vi "Configure.vi"(0 "disk streaming in":refnum<class "Disk Streaming.lvclass">, 1 "actual host DMA buffer size (samples)":u32, 2 "actual host DMA buffer size (elements)":u32, 3 "transfer quantum size (samples)":u64, 4 "sample count (-1)":i64=-1, 5 "error in (no error)":errorcluster, 6 "coerce sample count? (T)":bool=TRUE, 7 "reserve file size (F)":bool, 8 "record count (1)":i64=1, 9 "max operations":u32, 11 "timeout (5 s)":dbl=5.0) -> (13 "actual max operations":u32, 14 "disk streaming out":refnum<class "Disk Streaming.lvclass">, 15 "file allocation size (bytes)":u64, 16 "file size (samples)":i64, 18 "sample count out":i64, 19 "error out":errorcluster)   [LabVIEW 2021, in "Disk Streaming.lvclass"]
doc: "Configures the transfer parameters of the streaming between a disk and an FPGA Target. Open a TDMS file and create a disk streaming instance referencing the file for streaming samples between a disk and an FPGA Target using the <B>Open.vi</B>, then use this VI to configure the transfer. Use the <B>Get Next Transfer Size.vi</B> to get the size of the next block to transfer during the streaming process, then depending on the selected direction and the TDMS I/O functions, use the <B>Read (I16 Data Ref).vi</B>, <B>Read (I16).vi</B>, <B>Write (I16 Data Ref).vi</B> or <B>Write (I16).vi</B> to read or write the TDMS file. Use the <B>Configure Status.vi</B> to configure the streaming status properties. Use the <B>Get Status.vi</B> to get status information. Use the <B>Close.vi</B> to close the disk streaming instance and the TDMS file it uses.\n\nInputs:\n\n<B>disk streaming in</B>: Disk streaming instance input.\n\n<B>actual host DMA buffer size (samples)</B>: The size, in number of samples, of the host DMA buffer transferring the samples between the host and the FPGA Target.\n\n<B>actual host DMA buffer size (elements)</B>: The size, in number of elements, of the host DMA buffer transferring the samples between the host and the FPGA Target.\n\n<B>transfer quantum size (samples)</B>: The quantum size, in number of samples, supported by the FPGA Target when transferring samples between the host and the FPGA Target. The number of samples transferred in each block during the streaming is a multiple of this value.\n\n<B>sample count</B>, <B>record count</B>: The number of samples per record and the number of records to transfer during the streaming. Set any of these inputs to -1 for infinite streaming. When streaming to disk, use non-negative values on these inputs to configure a finite streaming to stream <B>record count</B> * <B>sample count</B> number of samples to disk. Similarly, when streaming from disk, a non-zero <B>sample count</B> value configures a finite streaming to stream <B>record count</B> * <B>sample count</B> samples from disk. When the end of file is reached during a stream from disk process, the file is reopened, and the file reading continues from the beginning of the file. When streaming from disk, a zero <B>sample count</B> value configures a finite streaming to stream until the end of file is reached <B>record count</B> times. The default value of the <B>sample count</B> input is -1, while the default value of the <B>record count</B> input is 1.\n\n<B>coerce sample count?</B>: If this input is true, then the <B>sample count</B> input will be rounded up to be a multiple of the device transfer quantum size and the disk transfer quantum size. The rounded value is returned on the <B>sample count out</B> output, and the VI will use the rounded value as the number of samples per record. The default value of this input is true.\n\n<B>reserve file size</B>: Set this input to true when streaming to disk to pre-allocate disk space for the TDMS file and to prevent fragmentation on a file-system level. The pre-allocation is only possible when performing a finite streaming to disk, otherwise this input is ignored. Note: on Windows systems with the User Account Control enabled the file pre-allocation requires to run LabVIEW or the application with administrator privileges to avoid a run-time error. The default value of this input is false.\n\n<B>max operations</B>: The maximum number of asynchronous reads or writes that can run simultaneously in the background. This VI uses an upper limit for this parameter which is the number of blocks that can fit into the host DMA buffer minus 1 (the value used on the <B># of blocks</B> input of the <B>Disk Streaming Open.vi</B> minus 1). If this input is less than 1, then the upper limit value is used instead, otherwise the value of this input is coerced between 1 and the upper limit. The default value of this input is 0.\n\n<B>timeout</B>: The timeout value, in seconds, for the TDMS asynchronous read or write functions. When the number of pending asynchronous operations reaches the maximum value, the TDMS asynchronous read or write function waits as long as the timeout value for a pending asynchronous operation to complete before issuing another asynchronous operation. If no asynchronous operation completes during the wait period, then the function returns a timeout error. The default value of this input is 5.\n\nOutputs:\n\n<B>disk streaming out</B>: Disk streaming instance output. Pass this output to the other Disk Streaming VIs to perform the streaming.\n\n<B>file allocation size (bytes)</B>: The number of bytes pre-allocated for the TDMS file. For large files of several terabytes, the operating system may take a significant amount of time to pre-allocate disk space. Insert a delay in your application after this VI to ensure the file size is fully reserved. For multiple files on separate RAID volumes, if you reserve the file size in a loop, insert a single delay after the loop to avoid serializing the delays. NI recommends a time delay of 500 ms/TB.\n\n<B>file size (samples)</B>: The number of samples used in the TDMS file. When streaming from disk this is the number of samples that is used from the TDMS file. When streaming to disk this is the number of samples that will be written into the TDMS file in case of a finite streaming, while in case of an infinite streaming to disk this output returns -1.\n\n<B>sample count out</B>: The actual number of samples per record that will be transferred during the streaming. In case of infinite streaming this output returns -1.\n\n<B>actual max operations</B>: The value selected as the maximum number of asynchronous reads or writes that can run simultaneously in the background."
uses:
  Disk Streaming.lvclass
  Disk Streaming.lvclass/Disk Streaming.ctl
  Private/Status.ctl
  IO mode.ctl
  <vilib>/Utility/error.llb/Error Cluster From Error Code.vi
  <vilib>/ErrorRing/Error Ring.xnode
  <vilib>/gmath/NI_Gmath.lvlib
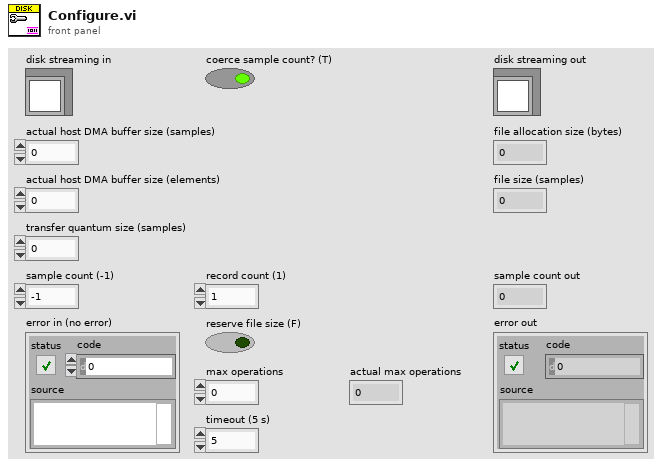
[diagram p1: front panel]
types:
  T1 = typedef "Disk Streaming.lvclass/IO mode.ctl" = enum16{"Synchronous", "Asynchronous", "Data Reference"}
  T2 = typedef "Disk Streaming.lvclass/Status.ctl" = cluster{"finished":bool, "Host DMA buffer size (bytes)":u64, "Host DMA buffer utilization (bytes)":u64, "Disk maximum async operations":u32, "Disk pending async operations":u32, "preview data":i16[]}
  T3 = typedef "Disk Streaming.lvclass/Data.ctl" = cluster{"tdms file":refnum<k34>, "group name":string, "channel name":string, "max operations":u32, "timeout (s)":dbl, "data type size (bytes)":u64, "writing":bool, "I/O mode":T1, "# of blocks":u32, "block size divisor (bytes)":u32, "file position (elements)":u64, "file size (elements)":i64, "file size (samples)":i64, "block size (elements)":u64, "block size (samples)":u64, "quantum size (elements)":u64, "quantum size (samples)":u64, "samples remaining":i64, "elements transferred":u64, "finished":bool, "preview size":i32, "preview quantum size (elements)":u64, "preview quantum size (samples)":u64, "DMA buffer size (elements)":u32, "pending block sizes (bytes)":u64[]}
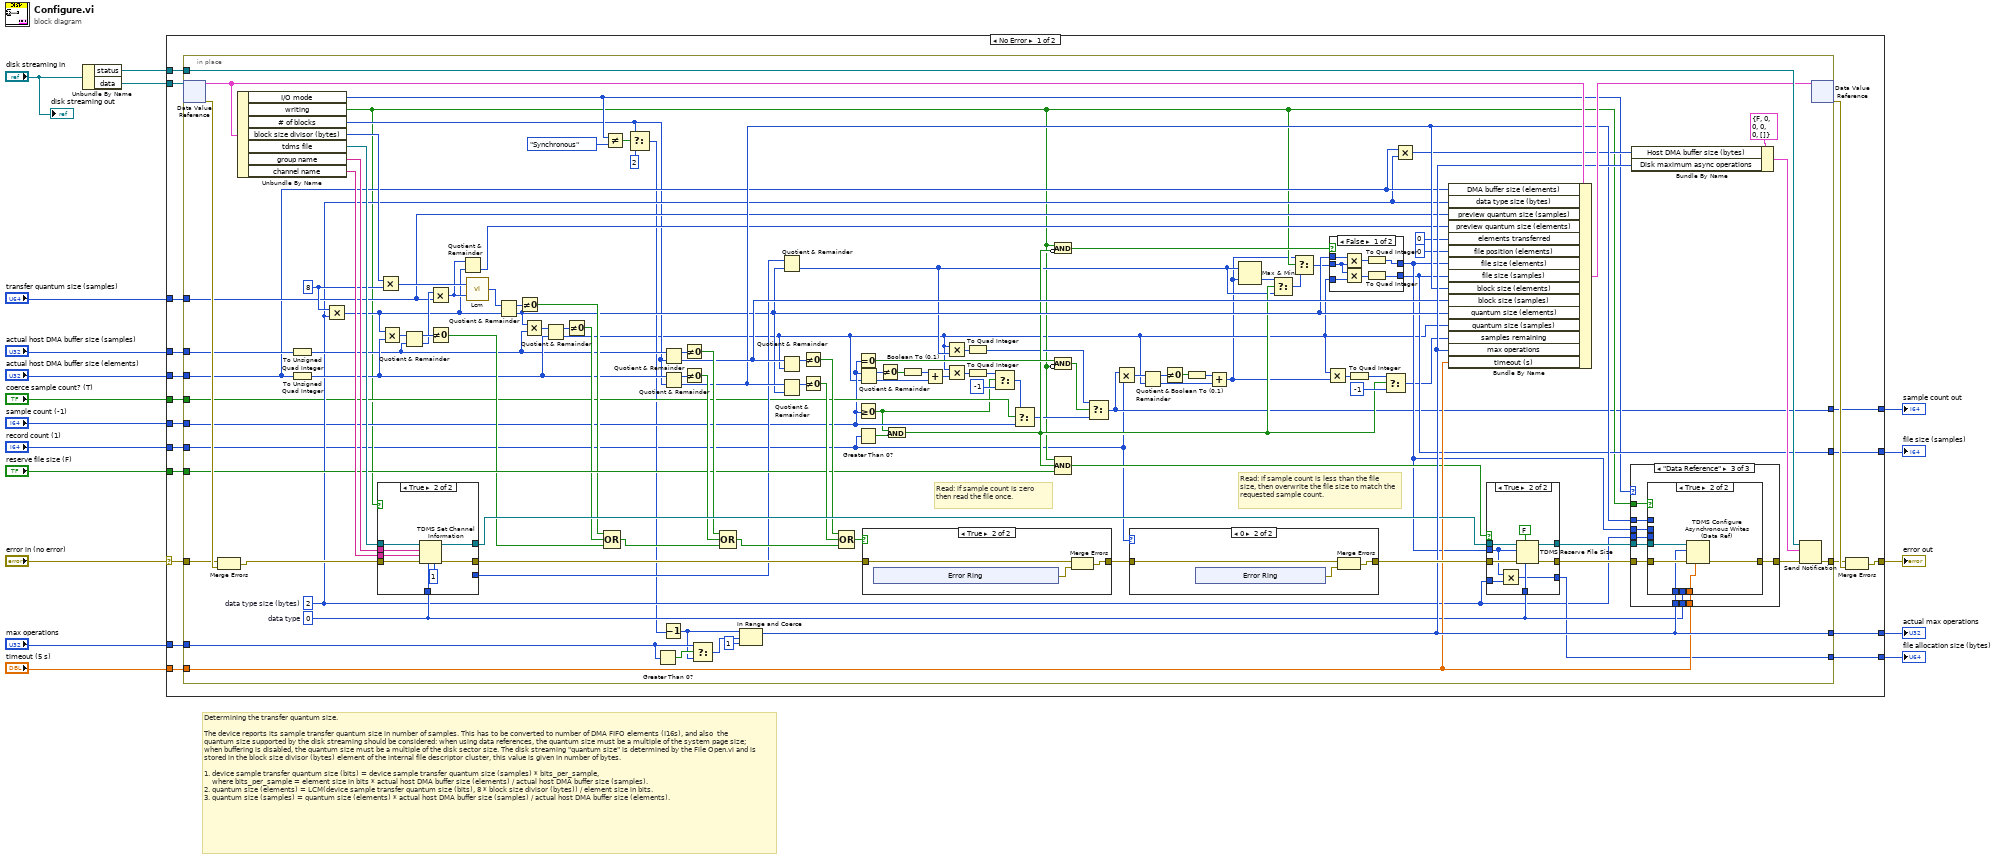
[diagram p0: block diagram]
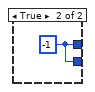
[diagram p3: hidden frame]
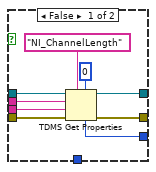
[diagram p4: hidden frame]
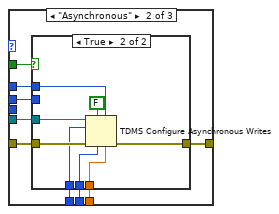
[diagram p6: hidden frame]
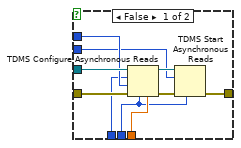
[diagram p7: hidden frame]
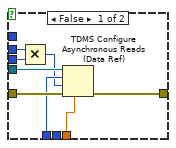
[diagram p8: hidden frame]
diagram:
  # "Determining the transfer quantum size.\n\nThe device reports its sample transfer quantum size in number of samples. This has to be converted to number of DMA FIFO elements (I16s), and also  the quantum size supported by the disk streaming should be considered: when using data references, the quantum size must be a multiple of the system page size; when buffering is disabled, the quantum size must be a multiple of the disk sector size. The disk streaming \"quantum size\" is determined by the File Open.vi and is stored in the block size divisor (bytes) element of the internal file descriptor cluster, this value is given in number of bytes.\n\n1. device sample transfer quantum size (bits) = device sample transfer quantum size (samples) * bits_per_sample,\n    where bits_per_sample = element size in bits * actual host DMA buffer size (elements) / actual host DMA buffer size (samples).\n2. quantum size (elements) = LCM(device sample transfer quantum size (bits), 8 * block size divisor (bytes)) / element size in bits.\n3. quantum size (samples) = quantum size (elements) * actual host DMA buffer size (samples) / actual host DMA buffer size (elements)."
  n1 = Unbundle By Name("disk streaming in") -> ("status"=w4:refnum<notifier>, "data"=w6:refnum<data-value>)
  n2 = case shown="No Error" "error in (no error)" {
    selector: "error in (no error)" -> [w36 w259]
    tunnel: [w34 w259] -> w17
    tunnel: "actual host DMA buffer size (samples)" -> [w33 _]
    tunnel: "actual host DMA buffer size (elements)" -> [w32 _]
    tunnel: "sample count (-1)" -> [w31 _]
    tunnel: "reserve file size (F)" -> [w30 _]
    tunnel: "max operations" -> [w29 _]
    tunnel: w6 -> [w28 _]
    tunnel: [w27 _] -> w11
    tunnel: "transfer quantum size (samples)" -> [w26 _]
    tunnel: "timeout (5 s)" -> [w25 _]
    tunnel: [w24 _] -> w8
    tunnel: [w23 _] -> w5
    tunnel: w4 -> [w22 _]
    tunnel: [w21 _] -> w3
    tunnel: "record count (1)" -> [w20 _]
    tunnel: "coerce sample count? (T)" -> [w19 _]
    frame No Error {
      n3 = in-place {
        in-place-border: w36 -> [w133]
        in-place-border: [w77] -> w35
        in-place-border: w33 -> [w124]
        in-place-border: w32 -> [w75]
        in-place-border: w31 -> [w63]
        in-place-border: w30 -> [w128]
        in-place-border: w29 -> [w91]
        in-place-border: [w46] -> w27
        in-place-border: w26 -> [w83]
        in-place-border: w25 -> [w141]
        in-place-border: [w147] -> w24
        in-place-border: [w79] -> w23
        in-place-border: w22 -> [w150]
        in-place-border: [w70] -> w21
        in-place-border: w20 -> [w38]
        in-place-border: w19 -> [w64]
        w95 = u64 8
        w74 = u64 2  # data type size (bytes)
        w96 = i16 0  # data type
        # "Read: if sample count is less than the file size, then overwrite the file size to match the requested sample count."
        # "Read: if sample count is zero then read the file once."
        n4 = in-place-dvr #1(w28) -> (w149:T3, w138:errorcluster)
        n5 = Merge Errors(w133, w138) -> (w110:errorcluster)
        n6 = Unbundle By Name(w149) -> ("I/O mode"=w68:T1, "writing"=w47:bool, "# of blocks"=w55:u32, "block size divisor (bytes)"=w127:u32, "tdms file"=w140:refnum<k34>, "group name"=w146:string, "channel name"=w145:string)
        n7 = To Unsigned Quad Integer(1:w124) -> (0:w86:u64)
        n8 = To Unsigned Quad Integer(1:w75) -> (0:w87:u64)
        n9 = Multiply(x=w95, y=w74) -> (x*y=w81:u64)
        n10 = case shown="True" w47 {
          tunnel: w110 -> [w175 w185]
          tunnel: w140 -> [w179 w187]
          tunnel: w145 -> [w177 w181]
          tunnel: w146 -> [w176 w182]
          tunnel: w96 -> [_ w183]
          tunnel: [w173 w184] -> w144
          tunnel: [w172 _] -> w106
          tunnel: [w178 w186] -> w143
          frame False {
            n11 = TDMS Get Properties(5:u64 0, 7:"NI_ChannelLength" ("property name"), 8:w175, 9:w177, 10:w176, 11:w179) -> (0:w173:errorcluster, 3:w178:refnum<k34>, 4:w172:u64)  [unwired: 3 out]
          }
          frame True {
            n12 = TDMS Set Channel Information(4:u32 1 ("samples per channel"), 6:w183, 8:w185, 9:w181, 10:w182, 11:w187) -> (0:w184:errorcluster, 3:w186:refnum<k34>)  [unwired: 1 in]
          }
        }
        n13 = Multiply(x=w127, y=w95) -> (x*y=w126:u64)
        n14 = Multiply(x=w81, y=w87) -> (x*y=w85:u64)
        n15 = Quotient & Remainder(x=w85, y=w86) -> (x-y*floor(x/y)=w122:u64, floor(x/y)=w84:u64)
        n16 = Multiply(x=w84, y=w83) -> (x*y=w82:u64)
        n17 = Not Equal To 0?(x=w122) -> (x != 0?=w109:bool)
        n18 = Quotient & Remainder(x=w82, y=w81) -> (floor(x/y)=w80:u64)  [unwired: 1 out]
        n19 = call <vilib>:"Lcm.vi"("y"=w82, "x"=w126) -> ("lcm(x,y)"=w125:i64)
        n20 = Quotient & Remainder(x=w125, y=w81) -> (x-y*floor(x/y)=w121:u64, floor(x/y)=w105:u64)
        n21 = Not Equal To 0?(x=w121) -> (x != 0?=w108:bool)
        n22 = Multiply(x=w105, y=w86) -> (x*y=w123:u64)
        n23 = Quotient & Remainder(x=w123, y=w87) -> (x-y*floor(x/y)=w120:u64, floor(x/y)=w40:u64)
        n24 = Not Equal To 0?(x=w120) -> (x != 0?=w107:bool)
        n25 = Compound Arithmetic op=OR(w108, w107, w109) -> (w117:bool)
        n26 = Not Equal?(x=w68, y=IO_mode."Synchronous") -> (x != y?=w66:bool)
        n27 = Select(t=w55, s=w66, f=u32 2) -> (s? t:f=w54:u32)
        n28 = Greater Than 0?(x=w91) -> (x > 0?=w92:bool)
        n29 = Decrement(x=w54) -> (x-1=w90:u32)
        n30 = Quotient & Remainder(x=w86, y=w55) -> (x-y*floor(x/y)=w119:u64, floor(x/y)=w116:u64)
        n31 = Quotient & Remainder(x=w87, y=w55) -> (x-y*floor(x/y)=w118:u64, floor(x/y)=w111:u64)
        n32 = Not Equal To 0?(x=w119) -> (x != 0?=w136:bool)
        n33 = Not Equal To 0?(x=w118) -> (x != 0?=w137:bool)
        n34 = Select(t=w91, s=w92, f=w90) -> (s? t:f=w89:u32)
        n35 = Compound Arithmetic op=OR(w136, w137, w117) -> (w113:bool)
        n36 = In Range and Coerce(upper limit=w90, x=w89, lower limit=u32 1) -> (coerced(x)=w147:u32)  [unwired: 1 out]
        n37 = Quotient & Remainder(x=w106, y=w105) -> (floor(x/y)=w51:u64)  [unwired: 1 out]
        n38 = Quotient & Remainder(x=w116, y=w40) -> (x-y*floor(x/y)=w115:u64)  [unwired: 1 out]
        n39 = Quotient & Remainder(x=w111, y=w105) -> (x-y*floor(x/y)=w114:u64)  [unwired: 1 out]
        n40 = Not Equal To 0?(x=w115) -> (x != 0?=w135:bool)
        n41 = Not Equal To 0?(x=w114) -> (x != 0?=w134:bool)
        n42 = Compound Arithmetic op=OR(w135, w134, w113) -> (w112:bool)
        n43 = Equal To 0?(x=w63) -> (x = 0?=w101:bool)
        n44 = Greater Or Equal To 0?(x=w63) -> (x >= 0?=w61:bool)
        n45 = Greater Than 0?(x=w38) -> (x > 0?=w62:bool)
        n46 = Quotient & Remainder(x=w63, y=w40) -> (x-y*floor(x/y)=w132:u64, floor(x/y)=w129:u64)
        n47 = case shown="True" w112 {
          tunnel: w144 -> [w239 w242]
          tunnel: [w239 w240] -> w153
          frame False {
          }
          frame True {
            n48 = xnode "Error Ring"() -> ("error out"=w241:errorcluster)
            n49 = Merge Errors(w242, w241) -> (w240:errorcluster)
          }
        }
        n50 = Not Equal To 0?(x=w132) -> (x != 0?=w131:bool)
        n51 = And(x=w61, y=w62) -> (x .and. y?=w56:bool)
        n52 = Boolean To (0,1)(Boolean=w131) -> (0, 1=w130:i16)
        n53 = Add(x=w130, y=w129) -> (x+y=w53:u64)
        n54 = Multiply(x=w40, y=w51) -> (x*y=w50:u64)
        n55 = Multiply(x=w40, y=w53) -> (x*y=w52:u64)
        n56 = To Quad Integer(1:w50) -> (0:w48:i64)
        n57 = To Quad Integer(1:w52) -> (0:w99:i64)
        n58 = Select(t=w99, s=w61, f=i64 -1) -> (s? t:f=w65:i64)
        n59 = Select(t=w65, s=w64, f=w63) -> (s? t:f=w49:i64)
        n60 = Compound Arithmetic op=AND(w47, invert w56) -> (w102:bool)
        n61 = Compound Arithmetic op=AND(w101, invert w47) -> (w100:bool)
        n62 = Compound Arithmetic op=AND(w47, w56, w128) -> (w139:bool)
        n63 = Select(t=w48, s=w100, f=w49) -> (s? t:f=w46:i64)
        n64 = Multiply(x=w46, y=w38) -> (x*y=w41:i64)
        n65 = case shown="0" w38 {
          tunnel: w153 -> [w154 w157]
          tunnel: [w154 w155] -> w152
          frame Default {
          }
          frame 0 {
            n66 = xnode "Error Ring"() -> ("error out"=w156:errorcluster)
            n67 = Merge Errors(w157, w156) -> (w155:errorcluster)
          }
        }
        n68 = Quotient & Remainder(x=w41, y=w40) -> (x-y*floor(x/y)=w42:u64, floor(x/y)=w45:u64)
        n69 = Not Equal To 0?(x=w42) -> (x != 0?=w43:bool)
        n70 = Boolean To (0,1)(Boolean=w43) -> (0, 1=w44:i16)
        n71 = Add(x=w44, y=w45) -> (x+y=w39:u64)
        n72 = Max & Min(x=w51, y=w39) -> (min(x,y)=w72:u64)  [unwired: 1 out]
        n73 = Select(t=w72, s=w56, f=w51) -> (s? t:f=w71:u64)
        n74 = Select(t=w39, s=w47, f=w71) -> (s? t:f=w104:u64)
        n75 = Multiply(x=w40, y=w39) -> (x*y=w58:u64)
        n76 = case shown="False" w102 {
          tunnel: w105 -> [w169 _]
          tunnel: w104 -> [w168 _]
          tunnel: w40 -> [w167 _]
          tunnel: [w164 w170] -> w97
          tunnel: [w163 w170] -> w70
          frame False {
            n77 = Multiply(x=w169, y=w168) -> (x*y=w166:u64)
            n78 = Multiply(x=w168, y=w167) -> (x*y=w165:u64)
            n79 = To Quad Integer(1:w166) -> (0:w164:i64)
            n80 = To Quad Integer(1:w165) -> (0:w163:i64)
          }
          frame True {
            w170 = i64 -1
          }
        }
        n81 = To Quad Integer(1:w58) -> (0:w59:i64)
        n82 = Select(t=w59, s=w56, f=i64 -1) -> (s? t:f=w57:i64)
        n83 = Multiply(x=w75, y=w74) -> (x*y=w73:u64)
        n84 = Bundle By Name(cluster=w149, "DMA buffer size (elements)"=w75, "data type size (bytes)"=w74, "preview quantum size (samples)"=w83, "preview quantum size (elements)"=w80, "elements transferred"=u64 0, "file position (elements)"=u64 0, "file size (elements)"=w97, "file size (samples)"=w70, "block size (elements)"=w111, "block size (samples)"=w116, "quantum size (elements)"=w105, "quantum size (samples)"=w40, "samples remaining"=w57, "max operations"=w147, "timeout (s)"=w141) -> (w148:T3)
        n85 = case shown="True" w139 {
          tunnel: [w249 w258] -> w103
          tunnel: [w248 w257] -> w142
          tunnel: w96 -> [_ w256]
          tunnel: w152 -> [w248 w255]
          tunnel: w143 -> [w249 w254]
          tunnel: w97 -> [_ w251]
          tunnel: w74 -> [_ w252]
          tunnel: [_ w250] -> w79
          frame False {
          }
          frame True {
            n86 = Multiply(x=w251, y=w252) -> (x*y=w250:u64)
            n87 = TDMS Reserve File Size(6:w256, 7:FALSE ("append? (T)"), 8:w255, 10:w251, 11:w254) -> (0:w257:errorcluster, 3:w258:refnum<k34>)
          }
        }
        n88 = case shown="\"Data Reference\"" w68 {
          tunnel: w142 -> [w188 w197 w225]
          tunnel: [w188 w196 w224] -> w78
          tunnel: w103 -> [_ w194 w222]
          tunnel: w96 -> [_ w195 w223]
          tunnel: w111 -> [_ w193 w221]
          tunnel: w47 -> [_ w192 w220]
          tunnel: w97 -> [_ w191 w219]
          tunnel: w147 -> [_ w190 w218]
          tunnel: w141 -> [_ w189 w217]
          tunnel: w74 -> [_ _ w216]
          frame "Synchronous" {
          }
          frame "Asynchronous" {
            n89 = case shown="True" w192 {
              tunnel: w197 -> [w207 w215]
              tunnel: [w199 w214] -> w196
              tunnel: w195 -> [w201 w213]
              tunnel: w194 -> [w206 w212]
              tunnel: w190 -> [w204 w211]
              tunnel: w193 -> [w205 w209]
              tunnel: w189 -> [w203 w208]
              tunnel: w191 -> [w198 _]
              frame False {
                n90 = TDMS Configure Asynchronous Reads(4:w203, 6:w201, 8:w207, 9:w205, 10:w204, 11:w206) -> (0:w202:errorcluster, 3:w200:refnum<k34>)
                n91 = TDMS Start Asynchronous Reads(6:w201, 8:w202, 10:w198, 11:w200) -> (0:w199:errorcluster)  [unwired: 1 out]
              }
              frame True {
                n92 = TDMS Configure Asynchronous Writes(4:w208, 5:w209, 6:w213, 7:FALSE ("pre-allocate? (F)"), 8:w215, 10:w211, 11:w212) -> (0:w214:errorcluster)  [unwired: 1 out]
              }
            }
          }
          frame "Data Reference" {
            n93 = case shown="True" w220 {
              tunnel: w225 -> [w233 w238]
              tunnel: [w230 w237] -> w224
              tunnel: w223 -> [_ _]
              tunnel: w222 -> [w232 w236]
              tunnel: w218 -> [w229 w234]
              tunnel: w221 -> [_ _]
              tunnel: w217 -> [w231 w235]
              tunnel: w219 -> [w227 _]
              tunnel: w216 -> [w228 _]
              frame False {
                n94 = Multiply(x=w227, y=w228) -> (x*y=w226:u64)
                n95 = TDMS Configure Asynchronous Reads (Data Ref)(6:w231, 8:w233, 9:w226, 10:w229, 11:w232) -> (0:w230:errorcluster)  [unwired: 1 out]
              }
              frame True {
                n96 = TDMS Configure Asynchronous Writes (Data Ref)(6:w235, 8:w238, 10:w234, 11:w236) -> (0:w237:errorcluster)  [unwired: 1 out]
              }
            }
          }
        }
        n97 = Bundle By Name(cluster=T2 {"finished"=FALSE, "Host DMA buffer size (bytes)"=0, "Host DMA buffer utilization (bytes)"=0, "Disk maximum async operations"=0, "Disk pending async operations"=0, "preview data"=[]} ("Disk Streaming Descriptor Status"), "Host DMA buffer size (bytes)"=w73, "Disk maximum async operations"=w147) -> (w151:T2)
        n98 = Send Notification(notification=w151, notifier=w150, error in (no error)=w78) -> (error out=w77:errorcluster)  [unwired: 1 out]
        n99 = in-place-dvr #1(w148) -> (w37:errorcluster)  [unwired: 1 out]
      }
      n100 = Merge Errors(w35, w37) -> (w34:errorcluster)
    }
    frame Error {
    }
  }
  "error out" <- w17
  "sample count out" <- w11
  "actual max operations" <- w8
  "file allocation size (bytes)" <- w5
  "file size (samples)" <- w3
  "disk streaming out" <- "disk streaming in"
